vi "Acq Get Status.vi"(0 "session in":refnum<class "Digitizer Control.lvclass">, 5 "error in (no error)":errorcluster) -> (7 "FIFO size":u64[](array[numeric]), 9 "FIFO utilization":cluster{"lowest":u64, "highest":u64}[](array[cluster]), 11 "memory size":u64[](array[numeric]), 13 "memory utilization":cluster{"lowest":u64, "highest":u64}[](array[cluster]), 14 "session out":refnum<class "Digitizer Control.lvclass">, 15 "acquiring":bool[](array[boolean]), 16 "samples acquired":u64[](array[numeric]), 17 "elements to read":u64[](array[numeric]), 18 "overflow":bool[](array[boolean]), 19 "error out":errorcluster)   [LabVIEW 2021, in "Digitizer Control.lvclass"]
doc: "Returns the acquisition status.\n\nInputs:\n\n<B>session in</B>: The device session.\n\nOutputs:\n\n<B>session out</B>: The device session passed on the <B>session in</B> input.\n\n<B>acquiring</B>: Indicates if an acquisition is in progress. This output is an array, the n-th element corresponds to the n-th channel.\n\n<B>samples acquired</B>: The number of samples acquired since the acquisition was initiated (including the samples acquired in all the records in case of a multi-record acquisition). This output is an array, the n-th element corresponds to the n-th channel.\n\n<B>elements to read</B>: The number of elements to read from the host DMA buffer to fetch the samples acquired since the acquisition was initiated. This output is an array, the n-th element corresponds to the n-th channel.\n\n<B>overflow</B>: Indicates if a DSP overflow occurred since the acquisition was initiated (when calling this VI for the first time after the acquisition was initiated), or since the last time this VI was called (when calling this VI again without initiating a new acquisition). This output is an array, the n-th element corresponds to the n-th channel.\n\n<B>FIFO size</B>: The size, in bytes, of the device FIFO accepting the acquired samples. This output is valid only in case the transfer is already configured by the <B>Acq Configure Transfer.vi</B>. This output is an array, the n-th element corresponds to the n-th channel.\n\n<B>FIFO utilization</B>: The <B>lowest</B> and <B>highest</B> number of sample bytes waited in the device FIFO accepting the acquired samples since the acquisition was initiated (when calling this VI for the first time after the acquisition was initiated), or since the last time this VI was called (when calling this VI again without initiating a new acquisition). This output is an array, the n-th element corresponds to the n-th channel.\n\n<B>memory size</B>: The size, in bytes, of the device memory available for buffering the acquired samples. This output is valid only in case the transfer is already configured by the <B>Acq Configure Transfer.vi</B>. This output is an array, the n-th element corresponds to the n-th channel.\n\n<B>memory utilization</B>: The <B>lowest</B> and <B>highest</B> number of sample bytes waited in the device memory available for buffering the acquired samples since the acquisition was initiated (when calling this VI for the first time after the acquisition was initiated), or since the last time this VI was called (when calling this VI again without initiating a new acquisition). This output is an array, the n-th element corresponds to the n-th channel."
uses:
  Digitizer Control.lvclass
  Digitizer Control.lvclass/Digitizer Control.ctl
  <vilib>/Utility/error.llb/Error Cluster From Error Code.vi
  <vilib>/rvi/errors/niLvFpgaAdjustHostInterfaceError.vi
  <vilib>/rvi/interface/nirviReadWriteControl/nirviReadWriteControl.xnode
  <vilib>/ErrorRing/Error Ring.xnode
  <instrlib>/_niInstr/Streaming/v1/Host/niInstr Streaming v1 Host.lvlib
  NiFpgaLv.dll
  <vilib>/rvi/interface/Simulation/niFpgaSimulationCallBeginRW.vi
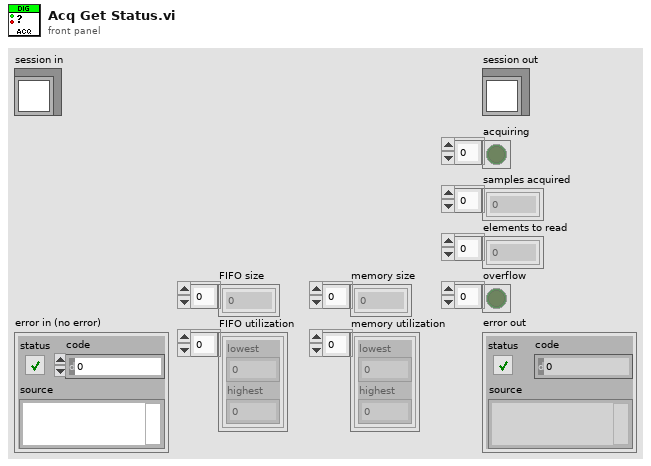
[diagram p1: front panel]
types:
  T1 = typedef "Digitizer Control.lvclass/Acq Session Data.ctl" = cluster{"ADC sampling rate":dbl, "SCTL rate":dbl, "DMA element size (bits)":i32, "sample size (bits)":i32[], "DMA/memory interface width (DMA elements)":i32, "transfer size (bits)":i32[], "stream instance":i32[], "trigger instance":u32, "group delay (s)":dbl, "data delay (s)":dbl, "target delay (s)":dbl, "trigger tracking enabled":bool, "channel configured":bool, "enabled channels":bool[], "transfer configured":bool, "dsp bypass":bool, "fractional decimator input rate":dbl, "fractional decimator output rate":dbl, "sample scale factor":dbl[], "memory size":u64[], "FIFO size":u64}
  T2 = typedef "niInstr Streaming v1 Common.lvlib/Stream State.ctl" = enum8{"Idle", "Finite Transfer", "Continuous", "Done", "Error", "Not Ready", "Cancel"}
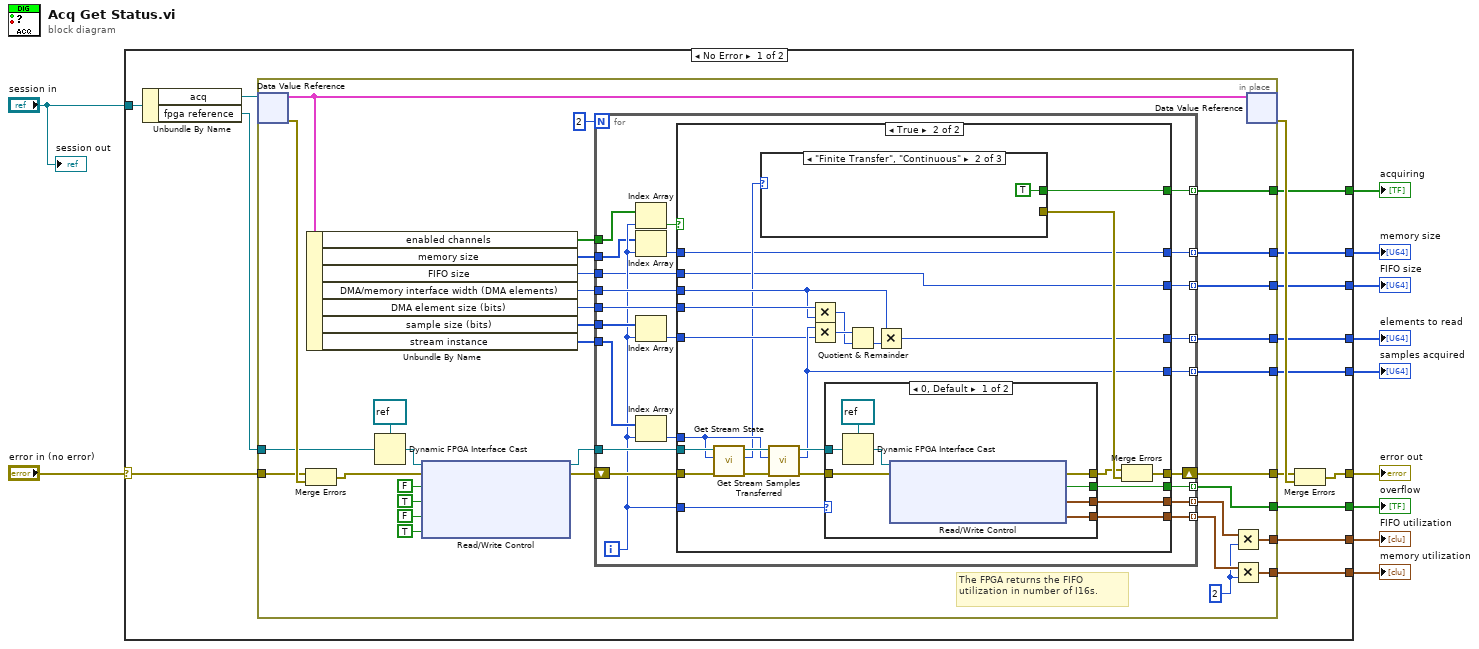
[diagram p0: block diagram]
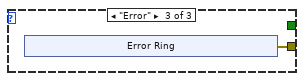
[diagram p4: hidden frame]
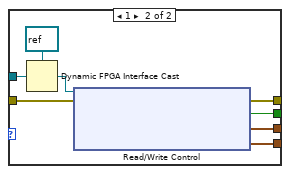
[diagram p5: hidden frame]
diagram:
  n1 = case shown="No Error" "error in (no error)" {
    selector: "error in (no error)" -> [w24 w133]
    tunnel: [w20 w133] -> w10
    tunnel: [w25 _] -> w9
    tunnel: [w23 _] -> w8
    tunnel: [w22 _] -> w7
    tunnel: "session in" -> [w16 _]
    tunnel: [w19 _] -> w6
    tunnel: [w18 _] -> w5
    tunnel: [w17 _] -> w4
    tunnel: [w13 _] -> w2
    tunnel: [w12 _] -> w1
    frame No Error {
      n2 = Unbundle By Name(w16) -> ("acq"=w15:refnum<data-value>, "fpga reference"=w14:refnum<k20>)
      n3 = in-place {
        in-place-border: [w58] -> w21
        in-place-border: [w57] -> w25
        in-place-border: w24 -> [w55]
        in-place-border: [w56] -> w23
        in-place-border: [w52] -> w22
        in-place-border: [w35] -> w19
        in-place-border: [w33] -> w18
        in-place-border: [w48] -> w17
        in-place-border: w14 -> [w46]
        in-place-border: [w28] -> w13
        in-place-border: [w27] -> w12
        w32 = u64 2
        # "The FPGA returns the FIFO utilization in number of I16s."
        n4 = in-place-dvr #1(w15) -> (w54:T1, w59:errorcluster)
        n5 = Merge Errors(w55, w59) -> (w45:errorcluster)
        n6 = Unbundle By Name(w54) -> ("enabled channels"=w31:bool[], "memory size"=w30:u64[], "FIFO size"=w29:u64, "DMA/memory interface width (DMA elements)"=w49:i32, "DMA element size (bits)"=w50:i32, "sample size (bits)"=w51:i32[], "stream instance"=w53:i32[])
        n7 = Dynamic FPGA Interface Cast(Session In=refnum<k20> refnum ("FPGA Interface"), Type=w46) -> (Session Out=w44:refnum<k20>)
        n8 = xnode "Read/Write Control"("FPGA VI Reference In"=w44, "error in"=w45, "acq.dsp.latch overflow"=FALSE, "acq.dsp.latch overflow"=TRUE, "acq.wfm.latch utilization"=FALSE, "acq.wfm.latch utilization"=TRUE) -> ("FPGA VI Reference Out"=w38:refnum<k20>, "error out"=w43:errorcluster)
        n9 = for {
          N: 2 -> [_]
          tunnel: [w81] -> w57 mode=indexing
          tunnel: [w80] -> w56 mode=indexing
          tunnel: w53 -> [w69]
          tunnel: [w79] -> w36 mode=indexing
          tunnel: [w78] -> w34 mode=indexing
          tunnel: [w77] -> w52 mode=indexing
          tunnel: w51 -> [w70]
          tunnel: w50 -> [w76]
          tunnel: w49 -> [w75]
          tunnel: [w74] -> w48 mode=indexing
          tunnel: w38 -> [w72]
          shift-right: [w82] -> w58
          shift-left: w43 -> [w73]
          tunnel: w31 -> [w71]
          tunnel: w30 -> [w64]
          tunnel: w29 -> [w62]
          tunnel: [w61] -> w28 mode=indexing
          tunnel: [w60] -> w27 mode=indexing
          i -> [w65]
          n10 = Index Array(array=w71, index=w65) -> (element=w67:bool)
          n11 = Index Array(array=w64, index=w65) -> (element=w63:u64)
          n12 = Index Array(array=w70, index=w65) -> (element=w66:i32)
          n13 = Index Array(array=w69, index=w65) -> (element=w68:i32)
          n14 = case shown="True" w67 {
            tunnel: [w83 w86] -> w82
            tunnel: [_ w105] -> w81
            tunnel: [_ w88] -> w80
            tunnel: [_ w102] -> w79
            tunnel: [_ w101] -> w78
            tunnel: [_ w100] -> w77
            tunnel: w76 -> [_ w98]
            tunnel: w75 -> [_ w96]
            tunnel: [_ w94] -> w74
            tunnel: w73 -> [w83 w93]
            tunnel: w72 -> [_ w107]
            tunnel: w68 -> [_ w92]
            tunnel: w65 -> [_ w91]
            tunnel: w66 -> [_ w90]
            tunnel: w63 -> [_ w85]
            tunnel: w62 -> [_ w84]
            tunnel: [_ w85] -> w61
            tunnel: [_ w84] -> w60
            frame False {
            }
            frame True {
              n15 = call <instrlib>:"Get Stream State.vi"("error in (no error)"=w93, "stream index"=w92, "refnum in"=w107) -> ("error out"=w104:errorcluster, "stream state"=w89:T2, "refnum out"=w108:refnum<k20>)  [unwired: 6 in]
              n16 = case shown="\"Finite Transfer\", \"Continuous\"" w89 {
                tunnel: [_ TRUE _] -> w88
                tunnel: [_ _ w111] -> w109
                frame Default {
                }
                frame "Finite Transfer", "Continuous" {
                }
                frame "Error" {
                  n17 = xnode "Error Ring"() -> ("error out"=w111:errorcluster)
                }
              }
              n18 = call <instrlib>:"Get Stream Samples Transferred.vi"("error in (no error)"=w104, "stream index"=w92, "refnum in"=w108) -> ("error out"=w103:errorcluster, "samples transferred"=w100:u64, "refnum out"=w106:refnum<k20>)  [unwired: 6 in]
              n19 = Multiply(x=w98, y=w96) -> (x*y=w97:i32)
              n20 = Multiply(x=w100, y=w90) -> (x*y=w99:u64)
              n21 = case shown="0, Default" w91 {
                tunnel: [w124 w132] -> w87
                tunnel: [w123 w131] -> w105
                tunnel: w103 -> [w122 w130]
                tunnel: [w121 w129] -> w102
                tunnel: [w120 w128] -> w101
                tunnel: w106 -> [w118 w126]
                frame 0, Default {
                  n22 = Dynamic FPGA Interface Cast(Session In=refnum<k20> refnum ("FPGA Interface"), Type=w118) -> (Session Out=w117:refnum<k20>)
                  n23 = xnode "Read/Write Control"("FPGA VI Reference In"=w117, "error in"=w122) -> ("error out"=w124:errorcluster, "acq.dsp.overflow 0"=w123:bool, "acq.wfm.FIFO utilization 0"=w121:cluster{"lowest":u32, "highest":u32}, "acq.wfm.memory utilization 0"=w120:cluster{"lowest":u32, "highest":u32})  [unwired: 1 out]
                }
                frame 1 {
                  n24 = Dynamic FPGA Interface Cast(Session In=refnum<k20> refnum ("FPGA Interface"), Type=w126) -> (Session Out=w125:refnum<k20>)
                  n25 = xnode "Read/Write Control"("FPGA VI Reference In"=w125, "error in"=w130) -> ("error out"=w132:errorcluster, "acq.dsp.overflow 1"=w131:bool, "acq.wfm.FIFO utilization 1"=w129:cluster{"lowest":u32, "highest":u32}, "acq.wfm.memory utilization 1"=w128:cluster{"lowest":u32, "highest":u32})  [unwired: 1 out]
                }
              }
              n26 = Quotient & Remainder(x=w99, y=w97) -> (floor(x/y)=w95:u64)  [unwired: 1 out]
              n27 = Multiply(x=w96, y=w95) -> (x*y=w94:u64)
              n28 = Merge Errors(w87, w109) -> (w86:errorcluster)
            }
          }
        }
        n29 = Multiply(x=w36, y=w32) -> (x*y=w35:cluster{"lowest":u64, "highest":u64}[])
        n30 = Multiply(x=w34, y=w32) -> (x*y=w33:cluster{"lowest":u64, "highest":u64}[])
        n31 = in-place-dvr #1(w54) -> (w26:errorcluster)  [unwired: 1 out]
      }
      n32 = Merge Errors(w21, w26) -> (w20:errorcluster)
    }
    frame Error {
    }
  }
  "error out" <- w10
  "overflow" <- w9
  "acquiring" <- w8
  "samples acquired" <- w7
  "FIFO utilization" <- w6
  "memory utilization" <- w5
  "elements to read" <- w4
  "memory size" <- w2
  "FIFO size" <- w1
  "session out" <- "session in"
